vi "Standard State Machine with Cleanup.vi"() -> ()   [LabVIEW 2011]
doc: "Use this template to build a standard state machine design pattern. Each state executes code and determines which state to transition to. Contrast this design pattern with the User Interface Event Handler pattern, in which code executes in response to user actions. Contrast this design pattern also with the Queued Message Handler pattern, in which each message handling code can queue zero or more new messages."
uses:
  Standard State Machine with Cleanup.ctl
panel:
  out "Elapsed Time (s)":dbl
  out "Stop":bool
  out "De-Initialize":bool
  out "Next Step":bool
  out "Initialize":bool
  in  "STOP":bool
  out "LED":bool
  out "Error":errorcluster
  # "1. LED will stay on after 5 seconds and do all steps beside De-Initialization before quiting"
  # "2. LED wil stay off and skip next step if stop button is pressed before 5 seconds \n    elapsed and will De-Initialize and quit"
  # "State Machine"
  # "Current State:"
  # "<- Next Step Turns LED On"
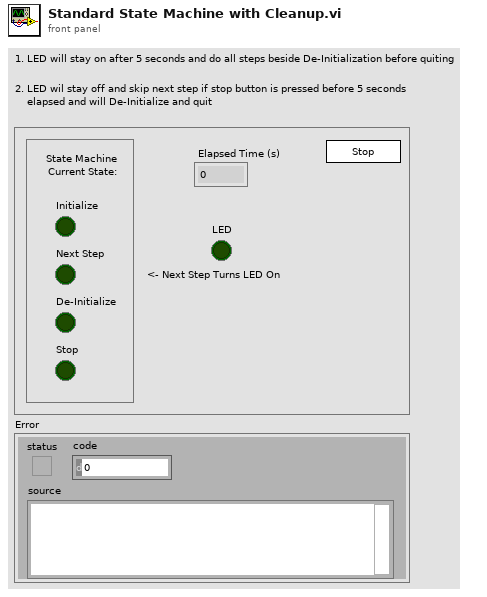
[diagram p1: front panel]
types:
  T1 = typedef "Standard State Machine with Cleanup.ctl" = enum16{"Initialize", "De-Initialize", "Next Step", "Stop"}
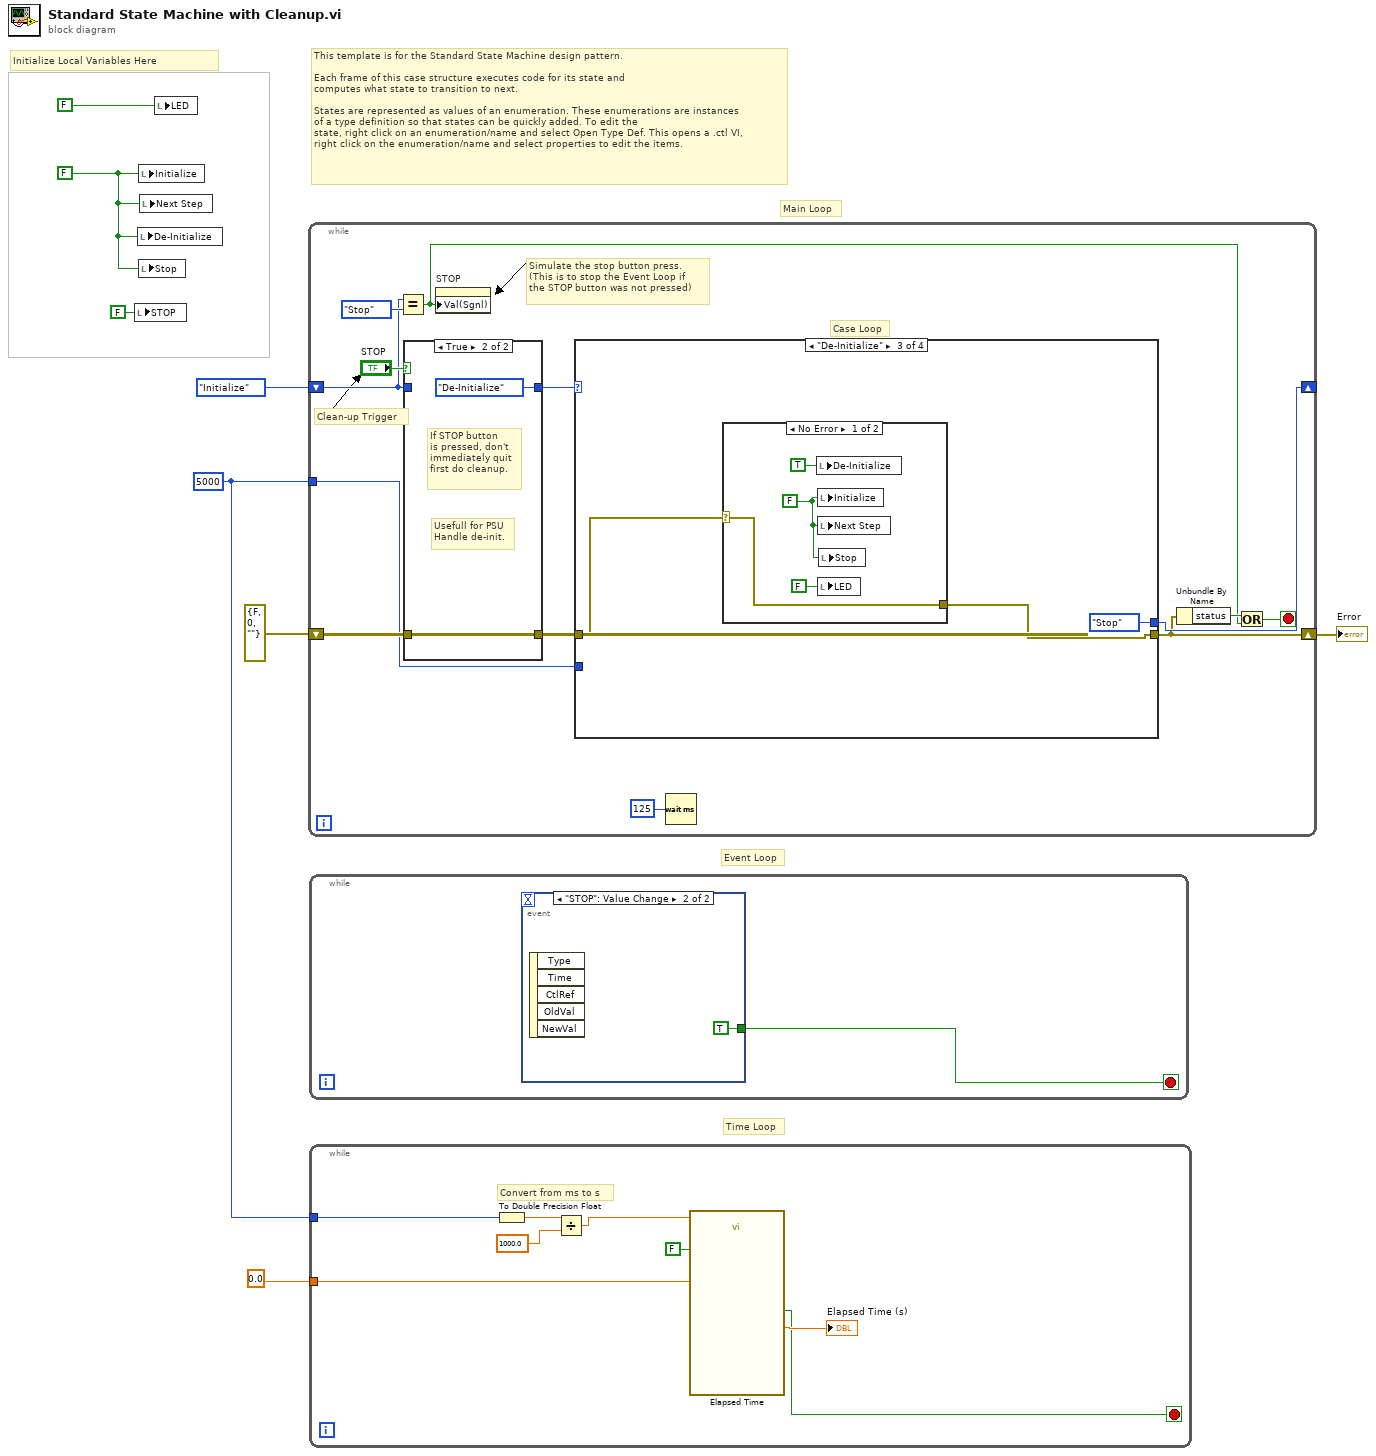
[diagram p0: block diagram]
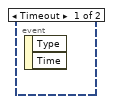
[diagram p2: hidden frame]
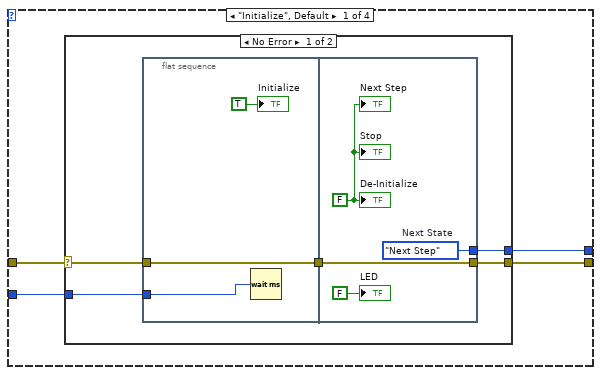
[diagram p4: hidden frame]
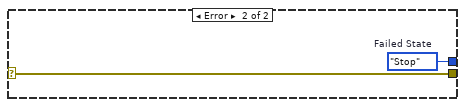
[diagram p5: hidden frame]
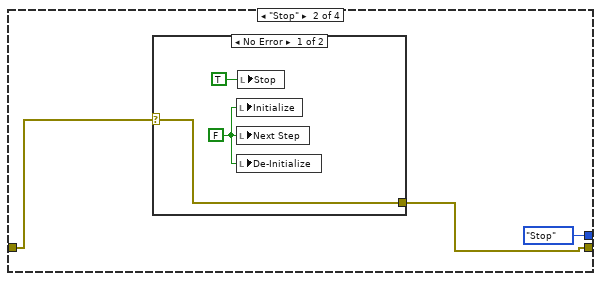
[diagram p6: hidden frame]
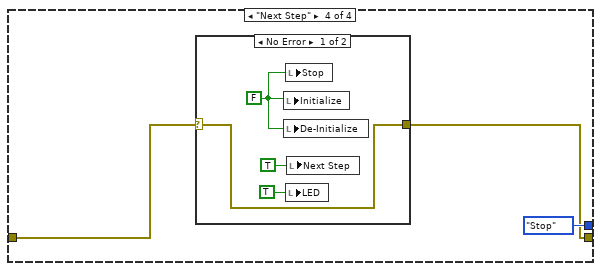
[diagram p9: hidden frame]
diagram:
  w2 = u32 5000 ("milliseconds to wait")
  w3 = FALSE ("Yeah!!")
  # "Time Loop"
  # "Event Loop"
  # "Main Loop"
  # "This template is for the Standard State Machine design pattern.\n\nEach frame of this case structure executes code for its state and\ncomputes what state to transition to next.\n\nStates are represented as values of an enumeration. These enumerations are instances\nof a type definition so that states can be quickly added. To edit the \nstate, right click on an enumeration/name and select Open Type Def. This opens a .ctl VI,\nright click on the enumeration/name and select properties to edit the items."
  # "Initialize Local Variables Here"
  n1 = local write "STOP"(FALSE ("STOP")) -> ()
  n2 = local write "De-Initialize"(w3) -> ()
  n3 = local write "Initialize"(w3) -> ()
  n4 = local write "Stop"(w3) -> ()
  n5 = local write "Next Step"(w3) -> ()
  n6 = local write "LED"(FALSE ("Yeah!!")) -> ()
  n7 = while {
    shift-right: [w15] -> _
    shift-left: Standard_State_Machine_with_Cleanup."Initialize" ("Next State") -> [w13]
    shift-right: [w14] -> w7
    shift-left: errorcluster {"status"=FALSE, "code"=0, "source"=""} ("error in (no error)") -> [w11]
    tunnel: w2 -> [w9]
    stop <- w19 stop-if-true
    # "Case Loop"
    # "Clean-up Trigger"
    # "Simulate the stop button press.\n(This is to stop the Event Loop if \nthe STOP button was not pressed)"
    n8 = Equal?(x=w13, y=Standard_State_Machine_with_Cleanup."Stop" ("States")) -> (x = y?=w17:bool)
    n9 = case shown="True" "STOP" {
      tunnel: [w22 w25] -> w10
      tunnel: w11 -> [w22 w25]
      tunnel: [w23 Standard_State_Machine_with_Cleanup."De-Initialize" ("Next State")] -> w12
      tunnel: w13 -> [w23 _]
      frame False {
      }
      frame True {
        # "Usefull for PSU\nHandle de-init."
        # "If STOP button\nis pressed, don't\nimmediately quit\nfirst do cleanup."
      }
    }
    n10 = property on="STOP" class="Bool (strict)"("Val(Sgnl)"=w17) -> ()  [unwired: 2 in, 2 out]
    n11 = case shown="\"De-Initialize\"" w12 {
      tunnel: [w27 Standard_State_Machine_with_Cleanup."Stop" ("Next State") Standard_State_Machine_with_Cleanup."Stop" ("Next State") Standard_State_Machine_with_Cleanup."Stop" ("Next State")] -> w15
      tunnel: w10 -> [w29 w45 w52 w60]
      tunnel: [w28 w44 w51 w59] -> w14
      tunnel: w9 -> [w26 _ _ _]
      frame "Initialize", Default {
        n12 = case shown="No Error" w29 {
          selector: w29 -> [w31 w43]
          tunnel: [w33 w43] -> w28
          tunnel: [w34 w42] -> w27
          tunnel: w26 -> [w30 _]
          frame No Error {
            n13 = flat-sequence {
              tunnel: [w37] -> w32
              tunnel: w31 -> [w37]
              tunnel: w30 -> [w35]
              tunnel: [w41] -> w34
              tunnel: [w38] -> w33
              tunnel: w32 -> [w38]
              frame #0 {
                n14 = Wait (ms)(milliseconds to wait=w35) -> ()  [unwired: 1 out]
                "Initialize" <- TRUE ("Initialize")
              }
              frame #1 {
                w40 = FALSE ("Stop")
                w41 = Standard_State_Machine_with_Cleanup."Next Step"  # Next State
                "Next Step" <- w40
                "De-Initialize" <- w40
                "Stop" <- w40
                "LED" <- FALSE ("LED")
              }
            }
          }
          frame Error {
            w42 = Standard_State_Machine_with_Cleanup."Stop"  # Failed State
          }
        }
      }
      frame "Stop" {
        n15 = case shown="No Error" w45 {
          selector: w45 -> [w47 w50]
          tunnel: [w47 w50] -> w44
          frame No Error {
            w48 = FALSE ("Stop")
            n16 = local write "Initialize"(w48) -> ()
            n17 = local write "Next Step"(w48) -> ()
            n18 = local write "De-Initialize"(w48) -> ()
            n19 = local write "Stop"(TRUE ("Initialize")) -> ()
          }
          frame Error {
          }
        }
      }
      frame "De-Initialize" {
        n20 = case shown="No Error" w52 {
          selector: w52 -> [w54 w58]
          tunnel: [w54 w58] -> w51
          frame No Error {
            w55 = FALSE ("Stop")
            n21 = local write "De-Initialize"(TRUE ("Initialize")) -> ()
            n22 = local write "Initialize"(w55) -> ()
            n23 = local write "Next Step"(w55) -> ()
            n24 = local write "LED"(FALSE ("Yeah!!")) -> ()
            n25 = local write "Stop"(w55) -> ()
          }
          frame Error {
          }
        }
      }
      frame "Next Step" {
        n26 = case shown="No Error" w60 {
          selector: w60 -> [w62 w66]
          tunnel: [w62 w66] -> w59
          frame No Error {
            w64 = FALSE ("Stop")
            n27 = local write "Initialize"(w64) -> ()
            n28 = local write "De-Initialize"(w64) -> ()
            n29 = local write "Stop"(w64) -> ()
            n30 = local write "LED"(TRUE ("Yeah!!")) -> ()
            n31 = local write "Next Step"(TRUE ("Initialize")) -> ()
          }
          frame Error {
          }
        }
      }
    }
    n32 = Wait (ms)(milliseconds to wait=u32 125) -> ()  [unwired: 1 out]
    n33 = Unbundle By Name(w14) -> ("status"=w18:bool)
    n34 = Or(x=w18, y=w17) -> (x .or. y?=w19:bool)
  }
  "Error" <- w7
  n35 = while {
    stop <- w67 stop-if-true
    n36 = event shown="[1] \"STOP\": Value Change" {
      selector: _ -> [_ _]
      dyn-events: _ -> [_ _]
      timeout: _ -> [_ _]
      tunnel: [_ TRUE ("NewVal")] -> w67
      event Timeout {
        n37 = event-data() -> ()  [unwired: 1 in, 2 out]
      }
      event "STOP": Value Change {
        n38 = event-data() -> ()  [unwired: 1 in, 5 out]
      }
    }
  }
  n39 = while {
    tunnel: w2 -> [w74]
    tunnel: 0.0 ("Set Start Time (s)") -> [w72]
    stop <- w75 stop-if-true
    # "Convert from ms to s"
    n40 = To Double Precision Float(number=w74) -> (double precision float=w71:dbl)
    n41 = Divide(x=w71, y=1000.0) -> (x/y=w69:dbl)
    n42 = call "Elapsed Time"("Time Target (s)"=w69, "Auto Reset"=FALSE, "Set Start Time (s)"=w72) -> ("Elapsed Time (s)"=→"Elapsed Time (s)":dbl, "Time has Elapsed"=w75:bool)  [unwired: 9 in, 6 out]
  }
